vi "PV ActiveLine - Continuous Output.vi"(7 "W/R":bool, 8 "Fehler (Eingang)":errorcluster, 9 "Continuous Mode":u8(ring) items=["100 ms", "1 s (default)", "1 minute"], 11 "Referenz in":refnum<visa-resource-name>) -> (0 "Cluster (Ausgang)":errorcluster, 3 "Referenz out":refnum<visa-resource-name>)   [LabVIEW 2013, in "PV ActiveLine.lvlib"]
doc: "COM - Continuous Output of Measurement Values (RS485)\n\nTransmit: COM [,a]\nReceive: b,sx.xxxxEsxx,c,sy.yyyyEsyy\n\nMode, a =\n0 –> 100 ms\n1 –> 1 s (default)\n2 –> 1 minute\n\nStatus gauge 1,\nb =\n0 –> Measurement data okay\n1 –> Underrange\n2 –> Overrange\n3 –> Sensor error\n4 –> Sensor off (IKR, PKR, IMR, PBR)\n5 –> No sensor (output: 5,2.0000E-2 [hPa])\n6 –> Identification error\n\n\nsx.xxxxEsxx = Measurement value gauge 1 1) [in current pressure unit]\n\nc= Status gauge 2\n\nsy.yyyyEsyy = Measurement value gauge 2 1) [in current pressure unit]\n\n\nValues always in exponential format. For logarithmic gauges, the 3rd and 4th decimal are always 0."
uses:
  <instrlib>/PV ActiveLine/PV ActiveLine.lvlib
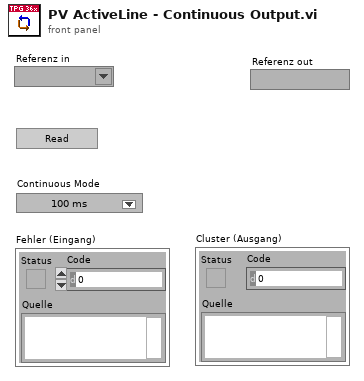
[diagram p1: front panel]
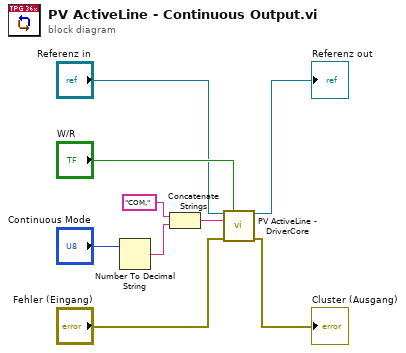
[diagram p0: block diagram]
diagram:
  n1 = Number To Decimal String(number="Continuous Mode") -> (decimal integer string=w5:string)  [unwired: 1 in]
  n2 = Concatenate Strings("COM,", w5) -> (w7:string)
  n3 = call <instrlib>:"PV ActiveLine - DriverCore.vi"("Referenz in"="Referenz in", "Write/Read"="W/R", "Command"=w7, "Fehler (Eingang)"="Fehler (Eingang)") -> ("Referenz out"=→"Referenz out":refnum<visa-resource-name>, "Cluster (Ausgang)"=→"Cluster (Ausgang)":errorcluster)  [unwired: 9 in, 1 out]
